vi "Initialize RF boards - with FPGA init only vi 16.3.1v1.vi"(2 "error in":errorcluster, 3 "FPGA Interface":T1) -> (0 "error out":errorcluster, 1 "FPGA Interface 2":T1)   [LabVIEW 2012]
uses:
  openfpgaref.initrf.ctl
  <vilib>/Utility/error.llb/Error Cluster From Error Code.vi
  <vilib>/rvi/errors/niLvFpgaAdjustHostInterfaceError.vi
  <vilib>/rvi/interface/nirviReadWriteControl/nirviReadWriteControl.xnode
  FPGA Bitfiles/UHR-FleezersInst_FPGATarget_intitializeRFsyn_v1.lvbitx
  NiFpgaLv.dll
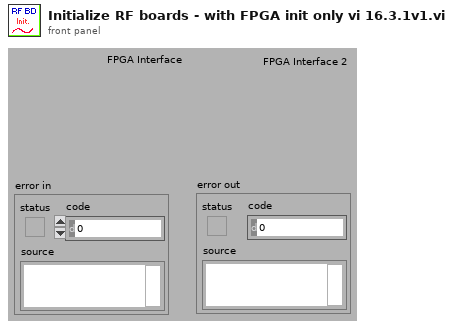
[diagram p1: front panel]
types:
  T1 = typedef "openfpgaref.initrf.ctl" = refnum<k20>
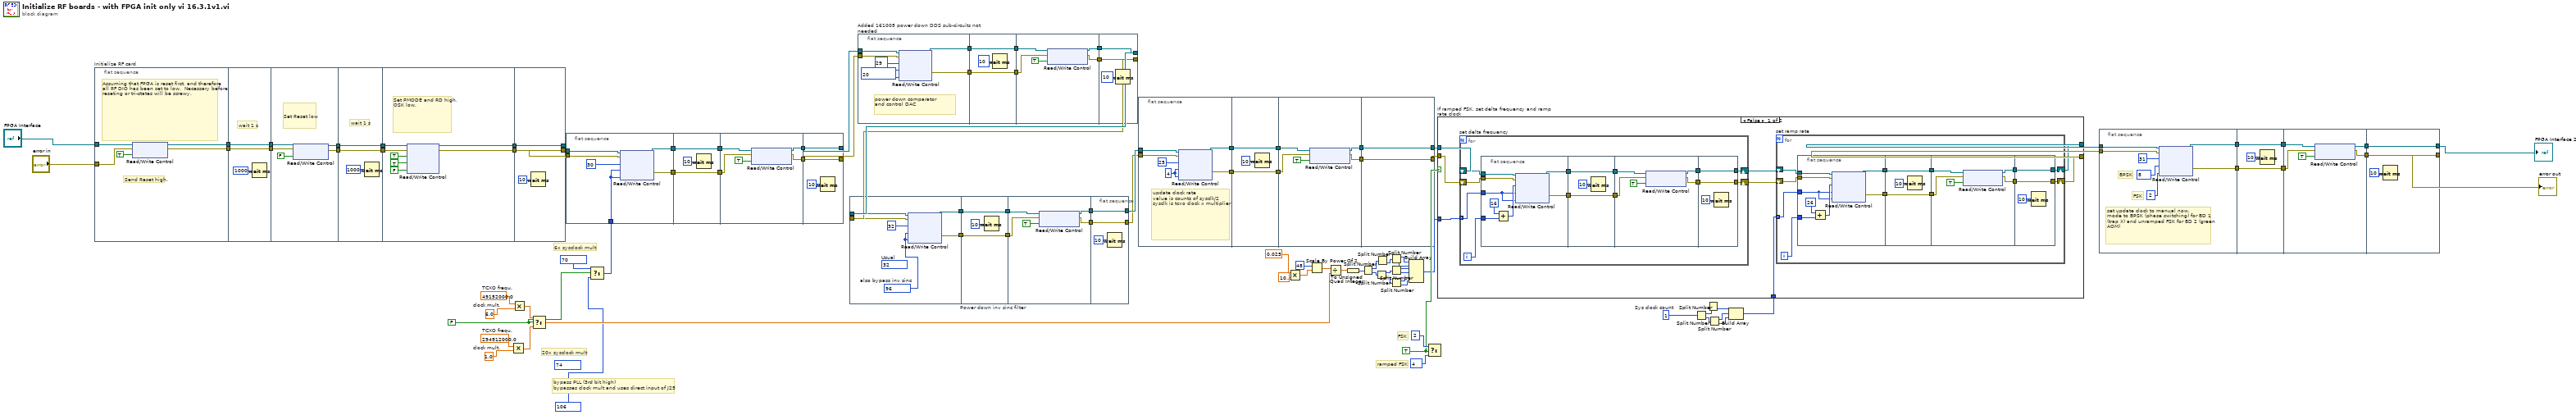
[diagram p0: block diagram]
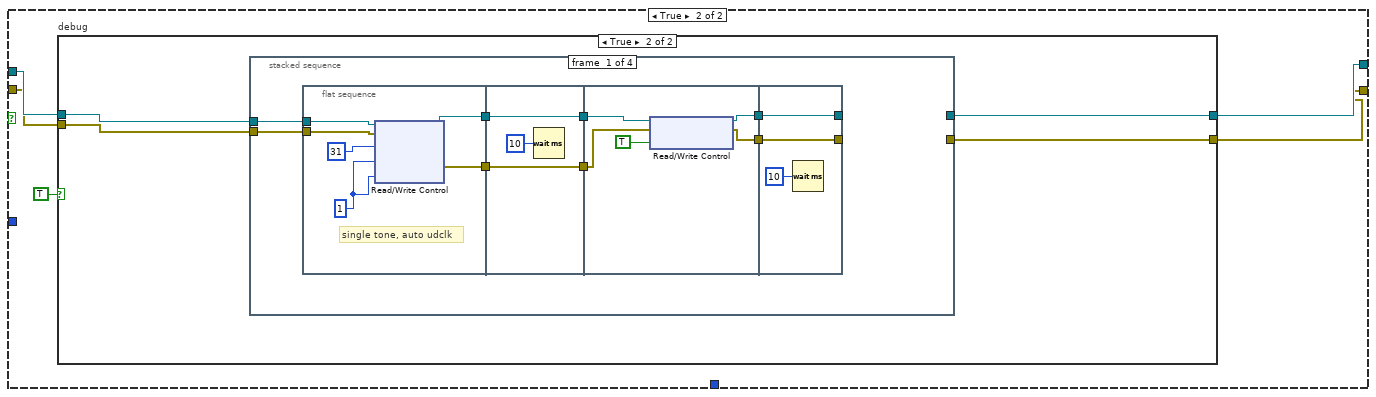
[diagram p2: hidden frame]
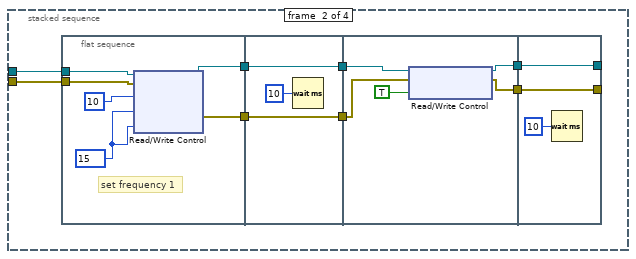
[diagram p4: hidden frame]
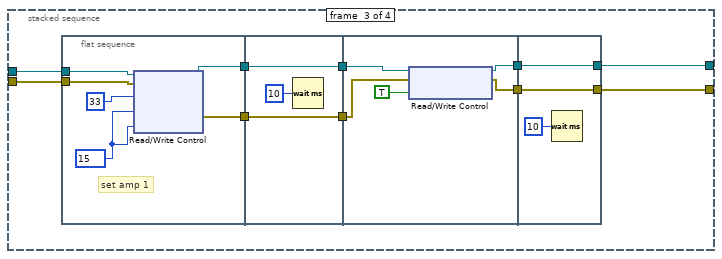
[diagram p5: hidden frame]
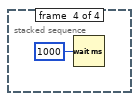
[diagram p6: hidden frame]
diagram:
  (unwired) u8 74 ("Data")
  w17 = FALSE ("s")
  w21 = 1.0  # clock mult.
  w20 = 294912000.0  # TCXO frequ.
  w24 = 6.0  # clock mult.
  w23 = 49152000.0  # TCXO frequ.
  w31 = u32 1  # Sys clock count
  w52 = TRUE
  # "bypass PLL (3rd bit high)\nbypasses clock mult and uses direct input of J25"
  # "20x sysclock mult"
  # "6x sysclock mult"
  # "ramped FSK"
  # "FSK"
  n1 = flat-sequence "Initialize RF card" {
    tunnel: [w101] -> w96
    tunnel: [w100] -> w95
    tunnel: "error in" -> [w99]
    tunnel: "FPGA Interface" -> [w97]
    tunnel: w96 -> [w103]
    tunnel: w95 -> [w102]
    tunnel: [w103] -> w94
    tunnel: [w102] -> w93
    tunnel: w94 -> [w109]
    tunnel: w93 -> [w108]
    tunnel: [w107] -> w92
    tunnel: [w106] -> w91
    tunnel: w92 -> [w111]
    tunnel: w91 -> [w110]
    tunnel: [w111] -> w90
    tunnel: [w110] -> w89
    tunnel: w90 -> [w119]
    tunnel: w89 -> [w118]
    tunnel: [w115] -> w79
    tunnel: [w114] -> w78
    tunnel: [w121] -> w72
    tunnel: [w122] -> w73
    tunnel: w79 -> [w122]
    tunnel: w78 -> [w121]
    frame #0 {
      # "Send Reset high."
      # "Assuming that FPGA is reset first, and therefore\nall RF DIO has been set to low.  Necessary before\nreseting or tri-states will be screwy."
      n2 = xnode "Read/Write Control"("FPGA VI Reference In"=w97, "error in"=w99, "Reset Bd 1"=TRUE ("Reset")) -> ("FPGA VI Reference Out"=w101:T1, "error out"=w100:errorcluster)
    }
    frame #1 {
      # "wait 1 s"
      n3 = Wait (ms)(milliseconds to wait=u32 1000) -> ()  [unwired: 1 out]
    }
    frame #2 {
      # "Set Reset low"
      n4 = xnode "Read/Write Control"("FPGA VI Reference In"=w109, "error in"=w108, "Reset Bd 1"=FALSE ("Reset")) -> ("FPGA VI Reference Out"=w107:T1, "error out"=w106:errorcluster)
    }
    frame #3 {
      # "wait 1 s"
      n5 = Wait (ms)(milliseconds to wait=u32 1000) -> ()  [unwired: 1 out]
    }
    frame #4 {
      # "Set PMODE and RD high,\nOSK low."
      n6 = xnode "Read/Write Control"("FPGA VI Reference In"=w119, "error in"=w118, "RD"=TRUE, "PMODE"=TRUE, "OSK Bd 1"=FALSE ("OSK")) -> ("FPGA VI Reference Out"=w115:T1, "error out"=w114:errorcluster)
    }
    frame #5 {
      n7 = Wait (ms)(milliseconds to wait=u32 10) -> ()  [unwired: 1 out]
    }
  }
  n8 = Multiply(x=w20, y=w21) -> (x*y=w19:dbl)
  n9 = Multiply(x=w23, y=w24) -> (x*y=w22:dbl)
  n10 = Select(t=w22, s=w17, f=w19) -> (s? t:f=w18:dbl)
  n11 = flat-sequence {
    tunnel: [w128] -> w88
    tunnel: [w127] -> w87
    tunnel: w73 -> [w126]
    tunnel: w72 -> [w125]
    tunnel: w15 -> [w123]
    tunnel: [w130] -> w86
    tunnel: w88 -> [w130]
    tunnel: [w129] -> w85
    tunnel: w87 -> [w129]
    tunnel: w86 -> [w136]
    tunnel: w85 -> [w135]
    tunnel: [w133] -> w77
    tunnel: [w132] -> w76
    tunnel: [w138] -> w6
    tunnel: [w139] -> w7
    tunnel: w77 -> [w139]
    tunnel: w76 -> [w138]
    frame #0 {
      n12 = xnode "Read/Write Control"("FPGA VI Reference In"=w126, "error in"=w125, "Address"=u8 30, "Data BD 1"=w123, "Data BD 2"=w123) -> ("FPGA VI Reference Out"=w128:T1, "error out"=w127:errorcluster)
    }
    frame #1 {
      n13 = Wait (ms)(milliseconds to wait=u32 10) -> ()  [unwired: 1 out]
    }
    frame #2 {
      n14 = xnode "Read/Write Control"("FPGA VI Reference In"=w136, "error in"=w135, "Update Data"=TRUE) -> ("FPGA VI Reference Out"=w133:T1, "error out"=w132:errorcluster)
    }
    frame #3 {
      n15 = Wait (ms)(milliseconds to wait=u32 10) -> ()  [unwired: 1 out]
    }
  }
  n16 = Select(t=u8 70 ("Data"), s=w17, f=u8 106 ("Data")) -> (s? t:f=w15:u8)
  n17 = flat-sequence "Power down inv sinc filter" {
    tunnel: [w145] -> w84
    tunnel: [w144] -> w83
    tunnel: w5 -> [w143]
    tunnel: w4 -> [w142]
    tunnel: [w147] -> w82
    tunnel: w84 -> [w147]
    tunnel: [w146] -> w81
    tunnel: w83 -> [w146]
    tunnel: w82 -> [w153]
    tunnel: w81 -> [w152]
    tunnel: [w150] -> w75
    tunnel: [w149] -> w74
    tunnel: [w155] -> w64
    tunnel: [w156] -> w65
    tunnel: w75 -> [w156]
    tunnel: w74 -> [w155]
    frame #0 {
      w140 = u8 96  # also bypass inv sinc
      (unwired) u8 32  # Usual
      n18 = xnode "Read/Write Control"("FPGA VI Reference In"=w143, "error in"=w142, "Address"=u8 32, "Data BD 1"=w140, "Data BD 2"=w140) -> ("FPGA VI Reference Out"=w145:T1, "error out"=w144:errorcluster)
    }
    frame #1 {
      n19 = Wait (ms)(milliseconds to wait=u32 10) -> ()  [unwired: 1 out]
    }
    frame #2 {
      n20 = xnode "Read/Write Control"("FPGA VI Reference In"=w153, "error in"=w152, "Update Data"=TRUE) -> ("FPGA VI Reference Out"=w150:T1, "error out"=w149:errorcluster)
    }
    frame #3 {
      n21 = Wait (ms)(milliseconds to wait=u32 10) -> ()  [unwired: 1 out]
    }
  }
  n22 = flat-sequence "Added 161005 power down DDS sub-circuits not needed" {
    tunnel: [w162] -> w13
    tunnel: [w161] -> w12
    tunnel: w7 -> [w160]
    tunnel: w6 -> [w159]
    tunnel: [w164] -> w11
    tunnel: w13 -> [w164]
    tunnel: [w163] -> w10
    tunnel: w12 -> [w163]
    tunnel: w11 -> [w170]
    tunnel: w10 -> [w169]
    tunnel: [w167] -> w9
    tunnel: [w166] -> w8
    tunnel: [w173] -> w4
    tunnel: w9 -> [w171]
    tunnel: w8 -> [w173]
    tunnel: [w171] -> w5
    frame #0 {
      w157 = u8 20 ("Data")
      # "power down comparator\nand control DAC"
      n23 = xnode "Read/Write Control"("FPGA VI Reference In"=w160, "error in"=w159, "Address"=u8 29, "Data BD 1"=w157, "Data BD 2"=w157) -> ("FPGA VI Reference Out"=w162:T1, "error out"=w161:errorcluster)
    }
    frame #1 {
      n24 = Wait (ms)(milliseconds to wait=u32 10) -> ()  [unwired: 1 out]
    }
    frame #2 {
      n25 = xnode "Read/Write Control"("FPGA VI Reference In"=w170, "error in"=w169, "Update Data"=TRUE) -> ("FPGA VI Reference Out"=w167:T1, "error out"=w166:errorcluster)
    }
    frame #3 {
      n26 = Wait (ms)(milliseconds to wait=u32 10) -> ()  [unwired: 1 out]
    }
  }
  n27 = flat-sequence {
    tunnel: [w179] -> w71
    tunnel: [w178] -> w70
    tunnel: w65 -> [w177]
    tunnel: w64 -> [w176]
    tunnel: [w181] -> w69
    tunnel: w71 -> [w181]
    tunnel: [w180] -> w68
    tunnel: w70 -> [w180]
    tunnel: w69 -> [w187]
    tunnel: w68 -> [w186]
    tunnel: [w184] -> w67
    tunnel: [w183] -> w66
    tunnel: [w188] -> w62
    tunnel: [w189] -> w63
    tunnel: w67 -> [w189]
    tunnel: w66 -> [w188]
    frame #0 {
      w174 = u8 4 ("Data")
      # "update clock rate\nvalue is counts of sysclk/2\nsysclk is tcxo clock x multiplier"
      n28 = xnode "Read/Write Control"("FPGA VI Reference In"=w177, "error in"=w176, "Address"=u8 25, "Data BD 1"=w174, "Data BD 2"=w174) -> ("FPGA VI Reference Out"=w179:T1, "error out"=w178:errorcluster)
    }
    frame #1 {
      n29 = Wait (ms)(milliseconds to wait=u32 10) -> ()  [unwired: 1 out]
    }
    frame #2 {
      n30 = xnode "Read/Write Control"("FPGA VI Reference In"=w187, "error in"=w186, "Update Data"=TRUE) -> ("FPGA VI Reference Out"=w184:T1, "error out"=w183:errorcluster)
    }
    frame #3 {
    }
  }
  n31 = Multiply(x=0.025 ("Delta Frequency  (MHz)"), y=1000000.0) -> (x*y=w47:dbl)
  n32 = Scale By Power Of 2(n=48, x=w47) -> (x*2^n=w49:dbl)
  n33 = Divide(x=w49, y=w18) -> (x/y=w48:dbl)
  n34 = To Unsigned Quad Integer(1:w48) -> (0:w44:u64)
  n35 = Split Number(x=w44) -> (hi(x)=w43:u32, lo(x)=w42:u32)
  n36 = Split Number(x=w42) -> (hi(x)=w40:u16, lo(x)=w41:u16)
  n37 = Split Number(x=w43) -> (lo(x)=w39:u16)  [unwired: 1 out]
  n38 = Split Number(x=w39) -> (hi(x)=w38:u8, lo(x)=w37:u8)
  n39 = Split Number(x=w40) -> (hi(x)=w36:u8, lo(x)=w35:u8)
  n40 = Split Number(x=w41) -> (hi(x)=w34:u8, lo(x)=w33:u8)
  n41 = Build Array(w38, w37, w36, w35, w34, w33) -> (w32:u8[])
  n42 = Select(t=u8 2 ("Data"), s=w52, f=u8 4 ("Data")) -> ()  [unwired: 1 out]
  n43 = Split Number(x=w31) -> (hi(x)=w30:u16, lo(x)=w29:u16)
  n44 = Split Number(x=w30) -> (lo(x)=w28:u8)  [unwired: 1 out]
  n45 = Split Number(x=w29) -> (hi(x)=w27:u8, lo(x)=w26:u8)
  n46 = Build Array(w28, w27, w26) -> (w25:u8[])
  n47 = case "If ramped FSK, set delta frequency and ramp rate clock" shown="False" w52 {
    tunnel: w63 -> [w197 w264]
    tunnel: w62 -> [w196 w263]
    tunnel: [w191 w260] -> w59
    tunnel: [w192 w261] -> w58
    tunnel: w32 -> [w195 _]
    tunnel: w25 -> [w190 _]
    frame False {
      n48 = for "set delta frequency" {
        shift-right: [w231] -> w194
        shift-left: w197 -> [w234]
        shift-right: [w232] -> w193
        shift-left: w196 -> [w233]
        tunnel: w195 -> [w229] mode=indexing
        i -> [w230]
        n49 = flat-sequence {
          tunnel: [w248] -> w240
          tunnel: [w247] -> w239
          tunnel: w234 -> [w246]
          tunnel: w233 -> [w245]
          tunnel: w230 -> [w243]
          tunnel: w229 -> [w241]
          tunnel: [w250] -> w238
          tunnel: w240 -> [w250]
          tunnel: [w249] -> w237
          tunnel: w239 -> [w249]
          tunnel: w238 -> [w256]
          tunnel: w237 -> [w255]
          tunnel: [w253] -> w236
          tunnel: [w252] -> w235
          tunnel: [w259] -> w232
          tunnel: [w257] -> w231
          tunnel: w236 -> [w257]
          tunnel: w235 -> [w259]
          frame #0 {
            n50 = Add(x=u8 16 ("Address"), y=w243) -> (x+y=w242:i32)
            n51 = xnode "Read/Write Control"("FPGA VI Reference In"=w246, "error in"=w245, "Address"=w242, "Data BD 1"=w241, "Data BD 2"=w241) -> ("FPGA VI Reference Out"=w248:T1, "error out"=w247:errorcluster)
          }
          frame #1 {
            n52 = Wait (ms)(milliseconds to wait=u32 10) -> ()  [unwired: 1 out]
          }
          frame #2 {
            n53 = xnode "Read/Write Control"("FPGA VI Reference In"=w256, "error in"=w255, "Update Data"=TRUE) -> ("FPGA VI Reference Out"=w253:T1, "error out"=w252:errorcluster)
          }
          frame #3 {
            n54 = Wait (ms)(milliseconds to wait=u32 10) -> ()  [unwired: 1 out]
          }
        }
      }
      n55 = for "set ramp rate" {
        shift-right: [w200] -> w192
        shift-left: w194 -> [w203]
        shift-right: [w201] -> w191
        shift-left: w193 -> [w202]
        tunnel: w190 -> [w198] mode=indexing
        i -> [w199]
        n56 = flat-sequence {
          tunnel: [w217] -> w209
          tunnel: [w216] -> w208
          tunnel: w203 -> [w215]
          tunnel: w202 -> [w214]
          tunnel: w199 -> [w212]
          tunnel: w198 -> [w210]
          tunnel: [w219] -> w207
          tunnel: w209 -> [w219]
          tunnel: [w218] -> w206
          tunnel: w208 -> [w218]
          tunnel: w207 -> [w225]
          tunnel: w206 -> [w224]
          tunnel: [w222] -> w205
          tunnel: [w221] -> w204
          tunnel: [w228] -> w201
          tunnel: [w226] -> w200
          tunnel: w205 -> [w226]
          tunnel: w204 -> [w228]
          frame #0 {
            n57 = Add(x=u8 26 ("Address"), y=w212) -> (x+y=w211:i32)
            n58 = xnode "Read/Write Control"("FPGA VI Reference In"=w215, "error in"=w214, "Address"=w211, "Data BD 1"=w210, "Data BD 2"=w210) -> ("FPGA VI Reference Out"=w217:T1, "error out"=w216:errorcluster)
          }
          frame #1 {
            n59 = Wait (ms)(milliseconds to wait=u32 10) -> ()  [unwired: 1 out]
          }
          frame #2 {
            n60 = xnode "Read/Write Control"("FPGA VI Reference In"=w225, "error in"=w224, "Update Data"=TRUE) -> ("FPGA VI Reference Out"=w222:T1, "error out"=w221:errorcluster)
          }
          frame #3 {
            n61 = Wait (ms)(milliseconds to wait=u32 10) -> ()  [unwired: 1 out]
          }
        }
      }
    }
    frame True {
      n62 = case "debug" shown="True" TRUE {
        tunnel: w264 -> [w266 w270]
        tunnel: w263 -> [w265 w269]
        tunnel: [w266 w268] -> w261
        tunnel: [w265 w267] -> w260
        frame False {
        }
        frame True {
          n63 = stacked-sequence {
            tunnel: w270 -> [w272 w297 w324 _]
            tunnel: w269 -> [w271 w296 w323 _]
            tunnel: [_ _ w322 _] -> w268
            tunnel: [_ _ w321 _] -> w267
            frame #0 {
              n64 = flat-sequence {
                tunnel: [w284] -> w278
                tunnel: [w283] -> w277
                tunnel: w272 -> [w282]
                tunnel: w271 -> [w281]
                tunnel: [w286] -> w276
                tunnel: w278 -> [w286]
                tunnel: [w285] -> w275
                tunnel: w277 -> [w285]
                tunnel: w276 -> [w292]
                tunnel: w275 -> [w291]
                tunnel: [w289] -> w274
                tunnel: [w288] -> w273
                tunnel: [w295] -> _
                tunnel: [w293] -> _
                tunnel: w274 -> [w293]
                tunnel: w273 -> [w295]
                frame #0 {
                  w279 = u8 1 ("Data")
                  # "single tone, auto udclk"
                  n65 = xnode "Read/Write Control"("FPGA VI Reference In"=w282, "error in"=w281, "Address"=u8 31, "Data BD 1"=w279, "Data BD 2"=w279) -> ("FPGA VI Reference Out"=w284:T1, "error out"=w283:errorcluster)
                }
                frame #1 {
                  n66 = Wait (ms)(milliseconds to wait=u32 10) -> ()  [unwired: 1 out]
                }
                frame #2 {
                  n67 = xnode "Read/Write Control"("FPGA VI Reference In"=w292, "error in"=w291, "Update Data"=TRUE) -> ("FPGA VI Reference Out"=w289:T1, "error out"=w288:errorcluster)
                }
                frame #3 {
                  n68 = Wait (ms)(milliseconds to wait=u32 10) -> ()  [unwired: 1 out]
                }
              }
            }
            frame #1 {
              n69 = flat-sequence {
                tunnel: [w309] -> w303
                tunnel: [w308] -> w302
                tunnel: w297 -> [w307]
                tunnel: w296 -> [w306]
                tunnel: [w311] -> w301
                tunnel: w303 -> [w311]
                tunnel: [w310] -> w300
                tunnel: w302 -> [w310]
                tunnel: w301 -> [w317]
                tunnel: w300 -> [w316]
                tunnel: [w314] -> w299
                tunnel: [w313] -> w298
                tunnel: [w320] -> _
                tunnel: [w318] -> _
                tunnel: w299 -> [w318]
                tunnel: w298 -> [w320]
                frame #0 {
                  w304 = u8 15 ("Data")
                  # "set frequency 1"
                  n70 = xnode "Read/Write Control"("FPGA VI Reference In"=w307, "error in"=w306, "Address"=u8 10, "Data BD 1"=w304, "Data BD 2"=w304) -> ("FPGA VI Reference Out"=w309:T1, "error out"=w308:errorcluster)
                }
                frame #1 {
                  n71 = Wait (ms)(milliseconds to wait=u32 10) -> ()  [unwired: 1 out]
                }
                frame #2 {
                  n72 = xnode "Read/Write Control"("FPGA VI Reference In"=w317, "error in"=w316, "Update Data"=TRUE) -> ("FPGA VI Reference Out"=w314:T1, "error out"=w313:errorcluster)
                }
                frame #3 {
                  n73 = Wait (ms)(milliseconds to wait=u32 10) -> ()  [unwired: 1 out]
                }
              }
            }
            frame #2 {
              n74 = flat-sequence {
                tunnel: [w336] -> w330
                tunnel: [w335] -> w329
                tunnel: w324 -> [w334]
                tunnel: w323 -> [w333]
                tunnel: [w338] -> w328
                tunnel: w330 -> [w338]
                tunnel: [w337] -> w327
                tunnel: w329 -> [w337]
                tunnel: w328 -> [w344]
                tunnel: w327 -> [w343]
                tunnel: [w341] -> w326
                tunnel: [w340] -> w325
                tunnel: [w347] -> w321
                tunnel: [w345] -> w322
                tunnel: w326 -> [w345]
                tunnel: w325 -> [w347]
                frame #0 {
                  w331 = u8 15 ("Data")
                  # "set amp 1"
                  n75 = xnode "Read/Write Control"("FPGA VI Reference In"=w334, "error in"=w333, "Address"=u8 33, "Data BD 1"=w331, "Data BD 2"=w331) -> ("FPGA VI Reference Out"=w336:T1, "error out"=w335:errorcluster)
                }
                frame #1 {
                  n76 = Wait (ms)(milliseconds to wait=u32 10) -> ()  [unwired: 1 out]
                }
                frame #2 {
                  n77 = xnode "Read/Write Control"("FPGA VI Reference In"=w344, "error in"=w343, "Update Data"=TRUE) -> ("FPGA VI Reference Out"=w341:T1, "error out"=w340:errorcluster)
                }
                frame #3 {
                  n78 = Wait (ms)(milliseconds to wait=u32 10) -> ()  [unwired: 1 out]
                }
              }
            }
            frame #3 {
              n79 = Wait (ms)(milliseconds to wait=u32 1000) -> ()  [unwired: 1 out]
            }
          }
        }
      }
    }
  }
  n80 = flat-sequence {
    tunnel: [w355] -> w57
    tunnel: [w354] -> w56
    tunnel: w58 -> [w353]
    tunnel: w59 -> [w352]
    tunnel: [w357] -> w55
    tunnel: w57 -> [w357]
    tunnel: [w356] -> w54
    tunnel: w56 -> [w356]
    tunnel: w55 -> [w363]
    tunnel: w54 -> [w362]
    tunnel: [w360] -> w53
    tunnel: [w359] -> w2
    tunnel: [w366] -> w51
    tunnel: w53 -> [w366]
    tunnel: [w364] -> w1
    tunnel: w2 -> [w364]
    frame #0 {
      # "BPSK"
      # "FSK"
      # "set update clock to manual now,\nmode to BPSK (phase switching) for BD 1 (trap X) and unramped FSK for BD 2 (green AOM)"
      n81 = xnode "Read/Write Control"("FPGA VI Reference In"=w353, "error in"=w352, "Address"=u8 31, "Data BD 1"=u8 8 ("Data"), "Data BD 2"=u8 2 ("Data")) -> ("FPGA VI Reference Out"=w355:T1, "error out"=w354:errorcluster)
    }
    frame #1 {
      n82 = Wait (ms)(milliseconds to wait=u32 10) -> ()  [unwired: 1 out]
    }
    frame #2 {
      n83 = xnode "Read/Write Control"("FPGA VI Reference In"=w363, "error in"=w362, "Update Data"=TRUE) -> ("FPGA VI Reference Out"=w359:T1, "error out"=w360:errorcluster)
    }
    frame #3 {
      n84 = Wait (ms)(milliseconds to wait=u32 10) -> ()  [unwired: 1 out]
    }
  }
  "error out" <- w51
  "FPGA Interface 2" <- w1
